vi "test_psf_internal.vi"() -> ()   [LabVIEW 2020]
panel:
  out "GreenMaxZ":T1(plugin-control)
  in  "Experiment folder path OR Z-stack folder path":path
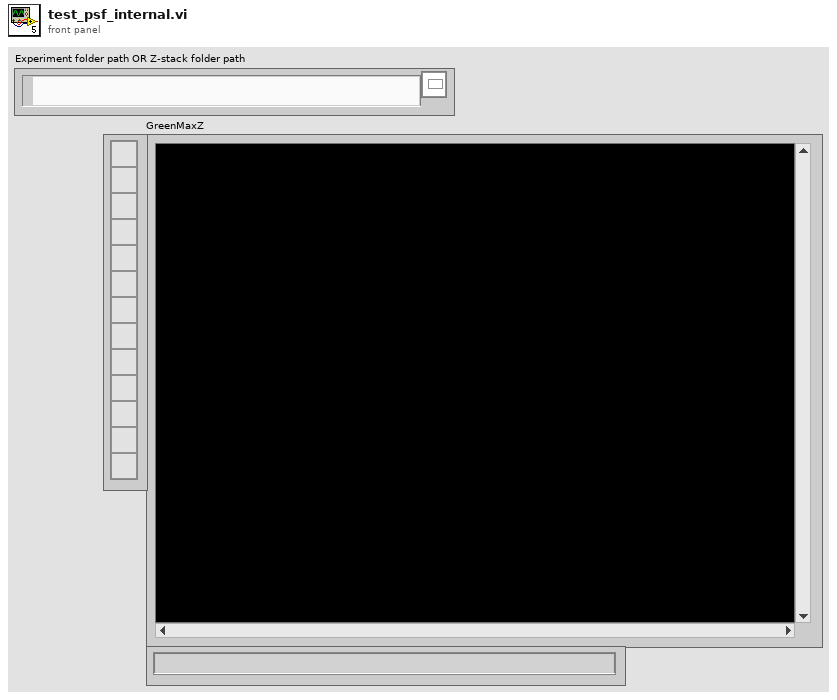
[diagram p1: front panel]
types:
  T1 = typedef "IMAQ Image.ctl" = refnum<image>
  T2 = cluster{"RedImageArray":T1[], "GreenImageArray":T1[], "RedMaxZ":T1, "GreenMaxZ":T1, "AOL Z Planes":dbl[], "AOL Z Planes (norm)":dbl[], "Motor Z planes":dbl[]}
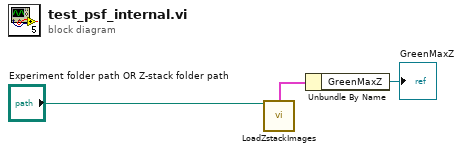
[diagram p0: block diagram]
diagram:
  n1 = call "LoadZstackImages.vi"("Experiment folder path OR Z-stack folder path"="Experiment folder path OR Z-stack folder path") -> ("All outputs"=w2:T2)  [unwired: 5 in, 9 out]
  n2 = Unbundle By Name(w2) -> ("GreenMaxZ"=→"GreenMaxZ":T1)
